vi "Update Dictionary.vi"(8 "error in (no error)":errorcluster, 9 "Variant":variant, 10 "Key":string, 11 "SMO.Dictionary.Variant in":refnum<class "SMO.Dictionary.Variant.lvclass">) -> (0 "error out":errorcluster, 3 "SMO.Dictionary.Variant out":refnum<class "SMO.Dictionary.Variant.lvclass">)   [LabVIEW 2013, in "SMO.Dictionary.lvlib" / "SMO.Dictionary.Variant.lvclass"]
uses:
  SMO.Dictionary.Variant.lvclass
  SMO.Dictionary.Variant.lvclass/SMO.Dictionary.Variant.ctl
  SMO.Dictionary/SMO.Dictionary.lvclass
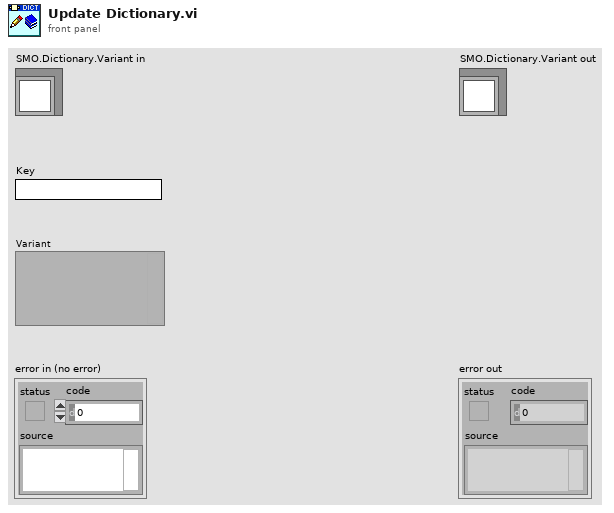
[diagram p1: front panel]
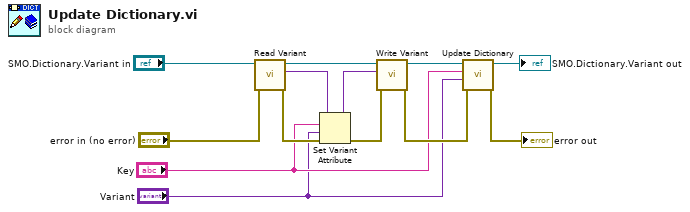
[diagram p0: block diagram]
diagram:
  n1 = call "Read Variant.vi"("error in (no error)"="error in (no error)", "SMO.Dictionary.Variant in"="SMO.Dictionary.Variant in") -> ("error out"=w7:errorcluster, "Variant"=w10:variant, "SMO.Dictionary.Variant out"=w13:refnum<class "SMO.Dictionary.Variant.lvclass">)  [unwired: 7 in]
  n2 = Set Variant Attribute(Variant=w10, name="Key", value="Variant", error in=w7) -> (Variant out=w11:variant, error out=w9:errorcluster)  [unwired: 1 out]
  n3 = call "Write Variant.vi"("error in (no error)"=w9, "Variant"=w11, "SMO.Dictionary.Variant in"=w13) -> ("error out"=w6:errorcluster, "SMO.Dictionary.Variant out"=w4:refnum<class "SMO.Dictionary.Variant.lvclass">)  [unwired: 7 in]
  n4 = call-parent "Update Dictionary.vi"("error in (no error)"=w6, "Variant"="Variant", "Key"="Key", "SMO.Dictionary in"=w4) -> ("error out"=→"error out":errorcluster, "SMO.Dictionary out"=→"SMO.Dictionary.Variant out":refnum<class "SMO.Dictionary.Variant.lvclass">)  [unwired: 6 in]
